vi "SMO.Dictionary.Update.vi"(6 "timeout (10ms)":i32=10, 8 "error in (no error)":errorcluster, 9 "Value":variant, 10 "Key (\"\": variant name)":string, 11 "SMO.Dictionary":refnum<class "SMO.Dictionary.lvclass">) -> (0 "error out":errorcluster, 3 "SMO.Dictionary out":refnum<class "SMO.Dictionary.lvclass">, 4 "timed out?":bool)   [LabVIEW 2013, in "SMO.Dictionary.lvlib" / "SMO.Dictionary.lvclass"]
doc: "---------------------------------------------------------------\nJKI State Machine Objects™\nhttp://jki.net/state-machine-objects/\nCopyright (C) 2005-2015, JKI <info@jki.net>\nALL RIGHTS RESERVEDJKI State Machine Objects (SMO) 1.0.0.4\nJKI - JKI\nCopyright (c) 2015, JKI"
uses:
  SMO.Dictionary.lvclass
  Typedefs/PrivateEvents--SMO.Dictionary.KeyValue-Pair.ctl
  <vilib>/Utility/VariantDataType/VariantType.lvlib
  <vilib>/JKI/JKI SMO/SMO/SMO.lvclass
panel:
  # "For instructions on how to use the JKI State Machine Objects, examples and video tutorials, visit:\nhttp://jki.net/state-machine-objects/\n\nJKI State Machine Objects™\nhttp://jki.net/state-machine-objects/\nCopyright (C) 2005-2015, JKI <info@jki.net>\nALL RIGHTS RESERVED"
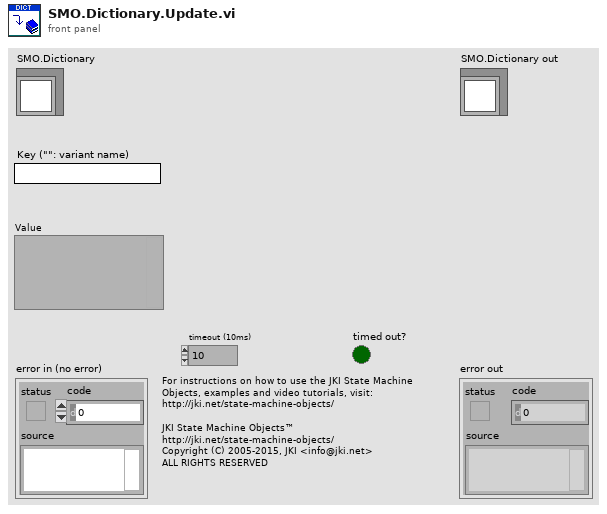
[diagram p1: front panel]
types:
  T1 = typedef "SMO.lvclass/SMOState --Enum.ctl" = enum16{"unknown", "Created", "Started", "Stopped"}
  T2 = typedef "SMO.Dictionary.lvlib/SMO.Dictionary.lvclass/PrivateEvents--SMO.Dictionary.KeyValue-Pair.ctl" = cluster{"Key":string, "Value":variant}
  T3 = typedef "SMO.Dictionary.lvlib/SMO.Dictionary.lvclass/PublicEvents--Cluster.ctl" = cluster{"Cleared":refnum<user-event>, "Deleted":refnum<user-event>, "Updated":refnum<user-event>}
  T4 = typedef "SMO.Dictionary.lvlib/SMO.Dictionary.lvclass/PrivateEvents--Cluster.ctl" = cluster{"Update":refnum<user-event>, "Clear Dictionary":refnum<user-event>, "Delete":refnum<user-event>, "Get":refnum<user-event>, "GetMultiple":refnum<user-event>}
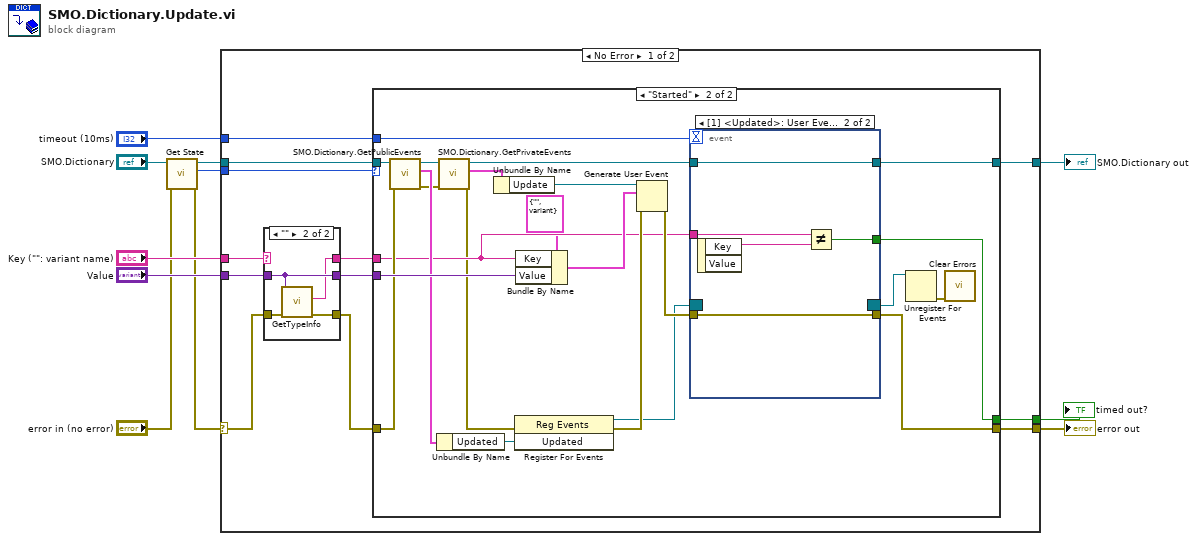
[diagram p0: block diagram]
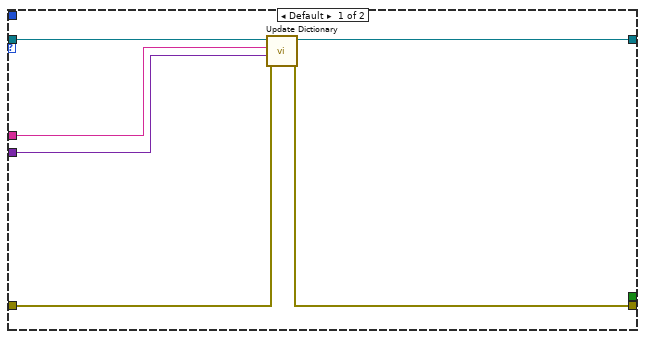
[diagram p3: hidden frame]
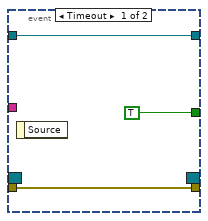
[diagram p4: hidden frame]
diagram:
  n1 = call <vilib>:"Get State.vi"("error in (no error)"="error in (no error)", "SMO"="SMO.Dictionary") -> ("error out"=w2:errorcluster, "SMO State"=w1:T1, "SMO out"=w4:refnum<class "SMO.Dictionary.lvclass">)  [unwired: 7 in]
  n2 = case shown="No Error" w2 {
    selector: w2 -> [w13 w69]
    tunnel: [w21 w69] -> w10
    tunnel: [w23 w68] -> w11
    tunnel: w4 -> [w19 w68]
    tunnel: "Key (\"\": variant name)" -> [w17 _]
    tunnel: "Value" -> [w16 _]
    tunnel: "timeout (10ms)" -> [w22 _]
    tunnel: [w20 _] -> w6
    tunnel: w1 -> [w18 _]
    frame No Error {
      n3 = case shown="\"\"" w17 {
        selector: w17 -> [w25 _]
        tunnel: w16 -> [w26 w30]
        tunnel: [w26 w30] -> w14
        tunnel: [w25 w29] -> w15
        tunnel: w13 -> [w24 w28]
        tunnel: [w24 w27] -> w12
        frame Default {
        }
        frame "" {
          n4 = call <vilib>:"GetTypeInfo.vi"("error in (no error)"=w28, "Variant"=w30) -> ("error out"=w27:errorcluster, "Name"=w29:string)  [unwired: 5 in, 3 out]
        }
      }
      n5 = case shown="\"Started\"" w18 {
        tunnel: w14 -> [w31 w57]
        tunnel: w15 -> [w32 w44]
        tunnel: w12 -> [w35 w53]
        tunnel: [w33 w49] -> w23
        tunnel: w22 -> [_ w42]
        tunnel: [w34 w47] -> w21
        tunnel: [_ w46] -> w20
        tunnel: w19 -> [w36 w54]
        frame Default {
          n6 = call-dynamic "Update Dictionary.vi"("error in (no error)"=w35, "Variant"=w31, "Key"=w32, "SMO.Dictionary in"=w36) -> ("error out"=w34:errorcluster, "SMO.Dictionary out"=w33:refnum<class "SMO.Dictionary.lvclass">)  [unwired: 6 in]
        }
        frame "Started" {
          n7 = call "SMO.Dictionary.GetPublicEvents.vi"("error in (no error)"=w53, "SMO.Dictionary in"=w54) -> ("error out"=w39:errorcluster, "Public Events"=w56:T3, "SMO.Dictionary out"=w41:refnum<class "SMO.Dictionary.lvclass">)  [unwired: 7 in]
          n8 = Unbundle By Name(w56) -> ("Updated"=w55:refnum<user-event>)
          n9 = call "SMO.Dictionary.GetPrivateEvents.vi"("error in (no error)"=w39, "SMO.Dictionary"=w41) -> ("error out"=w38:errorcluster, "Private Events"=w37:T4, "SMO.Dictionary out"=w40:refnum<class "SMO.Dictionary.lvclass">)  [unwired: 7 in]
          n10 = Unbundle By Name(w37) -> ("Update"=w59:refnum<user-event>)
          n11 = register-events(error in=w38, w55) -> (reference out=w45:refnum<event-registration>, error out=w52:errorcluster)  [unwired: 1 in]
          n12 = Bundle By Name(cluster=T2 {"Key"="", "Value"=variant} ("KVP"), "Key"=w44, "Value"=w57) -> (w58:T2)
          n13 = Generate User Event(user event=w59, event data cluster=w58, error in=w52) -> (error out=w48:errorcluster)  [unwired: 1 in, 1 out]
          n14 = event shown="[1] <Updated>: User Event" {
            selector: w45 -> [_ _]
            dyn-events: [_ _] -> w51
            timeout: w42 -> [_ _]
            tunnel: w40 -> [w62 w67]
            tunnel: [w62 w67] -> w49
            tunnel: w48 -> [w61 w66]
            tunnel: [w61 w66] -> w47
            tunnel: [TRUE w64] -> w46
            tunnel: w44 -> [_ w63]
            event Timeout {
              n15 = event-data() -> ()  [unwired: 1 in, 1 out]
            }
            event User Event {
              n16 = event-data() -> ("Key"=w65:string)  [unwired: 1 in, 1 out]
              n17 = Not Equal?(x=w63, y=w65) -> (x != y?=w64:bool)
            }
          }
          n18 = Unregister For Events(event registration refnum=w51) -> (error out=w50:errorcluster)  [unwired: 1 in]
          n19 = call <vilib>:"Clear Errors.vi"("error in (no error)"=w50) -> ()  [unwired: 6 in, 1 out]
        }
      }
    }
    frame Error {
    }
  }
  "error out" <- w10
  "SMO.Dictionary out" <- w11
  "timed out?" <- w6
